vi "array test.vi"() -> ()   [LabVIEW 2014]
panel:
  out "最后的数组":dbl[](array[numeric])
  out "二维数组大小":i32[](array[numeric])
  out "转置":dbl[][](array[numeric])
  out "数组":dbl[][](array[numeric])
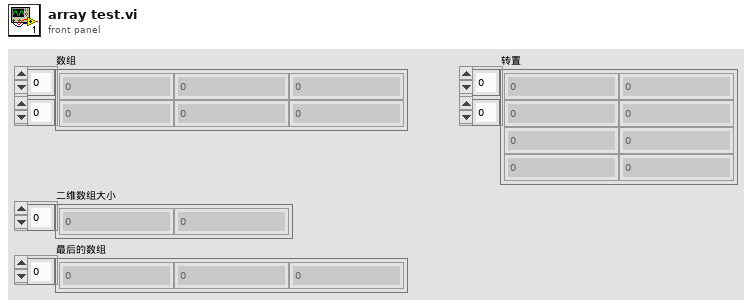
[diagram p1: front panel]
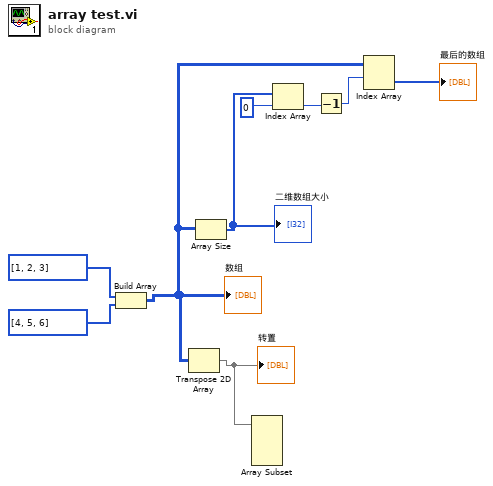
[diagram p0: block diagram]
diagram:
  n1 = Build Array(i32[] [1, 2, 3], i32[] [4, 5, 6]) -> (w6:i32[][])
  "数组" <- w6
  n2 = Transpose 2D Array(2D array=w6) -> (transposed array=w9:i32[][])
  "转置" <- w9
  n3 = Array Size(array=w6) -> (size(s)=w5:i32[])
  "二维数组大小" <- w5
  n4 = Array Subset(array=w9) -> ()  [unwired: 4 in, 1 out]
  n5 = Index Array(array=w5, index=0) -> (element=w3:i32)
  n6 = Decrement(x=w3) -> (x-1=w2:i32)
  n7 = Index Array(array=w6, index (row)=w2) -> (element=→"最后的数组":i32[])  [unwired: 1 in]
